vi "Handle Error.vi"(8 "error in (no error)":errorcluster, 11 "IMAQdx Actor in":refnum<class "IMAQdx Actor.lvclass">) -> (0 "error out":errorcluster, 2 "stop actor?":bool=TRUE, 3 "IMAQdx Actor out":refnum<class "IMAQdx Actor.lvclass">)   [LabVIEW 2014, in "IMAQdx Actor.lvlib" / "IMAQdx Actor.lvclass"]
doc: "(<B>Filename</B>: Actor Framework.lvlib:Actor.lvclass:Handle Error.vi)\n\nDefines how the actor handles an error that occurred while processing a message. By default, this method does nothing except stop the actor."
uses:
  IMAQdx Actor.lvclass
  Camera Actor/Camera Actor/Camera Actor.lvclass
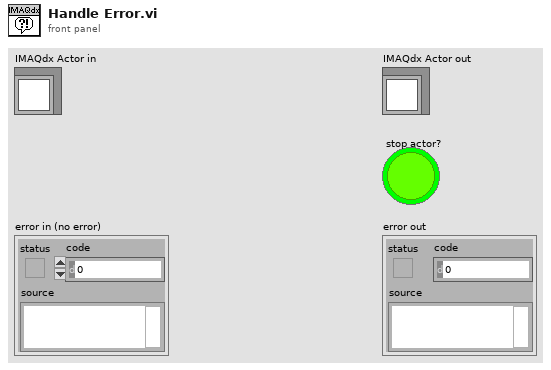
[diagram p1: front panel]
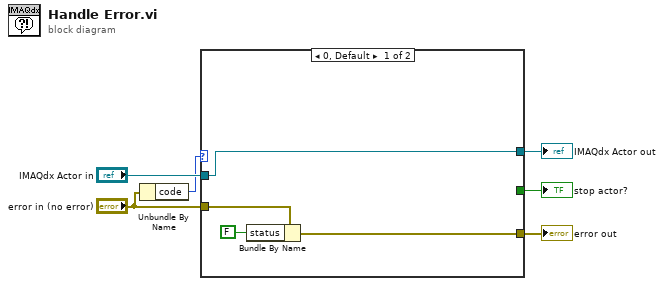
[diagram p0: block diagram]
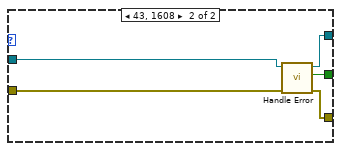
[diagram p2: hidden frame]
diagram:
  n1 = Unbundle By Name("error in (no error)") -> ("code"=w1:i32)
  n2 = case shown="0, Default" w1 {
    tunnel: [w9 w15] -> w6
    tunnel: [_ w14] -> w5
    tunnel: [w7 w13] -> w4
    tunnel: "error in (no error)" -> [w10 w12]
    tunnel: "IMAQdx Actor in" -> [w7 w11]
    frame 0, Default {
      n3 = Bundle By Name(cluster=w10, "status"=FALSE) -> (w9:errorcluster)
    }
    frame 43, 1608 {
      n4 = call-parent "Handle Error.vi"("error in (no error)"=w12, "IMAQdx Actor in"=w11) -> ("error out"=w15:errorcluster, "stop actor?"=w14:bool, "IMAQdx Actor out"=w13:refnum<class "IMAQdx Actor.lvclass">)  [unwired: 7 in]
    }
  }
  "IMAQdx Actor out" <- w4
  "error out" <- w6
  "stop actor?" <- w5
